vi "Num2littleEndian(DBL).vi"(7 "Number":dbl) -> (8 "LiitleEndianedData":u8[](array[numeric]))   [LabVIEW 2011]
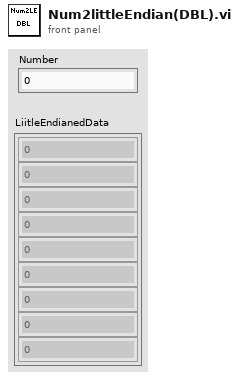
[diagram p1: front panel]
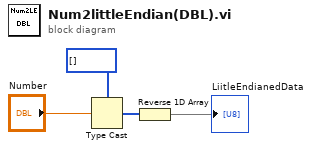
[diagram p0: block diagram]
diagram:
  n1 = Type Cast(type=u8[] [] ("initialized array"), x="Number") -> (*(type *) &x=w4:u8[])
  n2 = Reverse 1D Array(array=w4) -> (reversed array=→"LiitleEndianedData":u8[])
